vi "Find Subaddress.vi"(8 "error in":errorcluster, 10 "terminal subaddress":u16, 11 "remote terminal in":T1 format="%.0x") -> (0 "error out":errorcluster, 2 "subaddress":T1 format="%.0x", 3 "remote terminal out":T1 format="%.0x", 4 "found?":bool)   [LabVIEW 2020, in "Ballard MIL-STD-1553 Scripting.lvlib"]
uses:
  Ballard MIL-STD-1553 Scripting.lvlib
  <vilib>/NI VeriStand/Custom Device API/Custom Device Item Ref.ctl
  <vilib>/NI VeriStand/Custom Device API/Custom Device API.lvlib
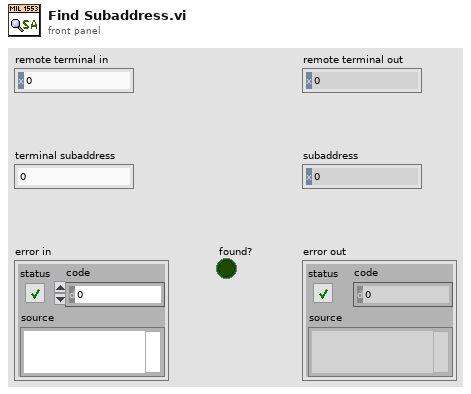
[diagram p1: front panel]
types:
  T1 = typedef "Custom Device API.lvlib/Custom Device Item Ref.ctl" = u64
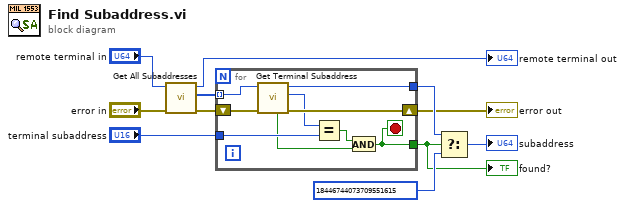
[diagram p0: block diagram]
diagram:
  n1 = call "Get All Subaddresses.vi"("error in"="error in", "remote terminal in"="remote terminal in") -> ("error out"=w6:errorcluster, "subaddresses"=w3:T1[], "remote terminal out"=→"remote terminal out":T1)  [unwired: 7 in]
  n2 = for {
    tunnel: w3 -> [w20] mode=indexing
    tunnel: "terminal subaddress" -> [w19]
    tunnel: [w14] -> w11
    tunnel: [w13] -> w2
    shift-right: [w15] -> w5
    shift-left: w6 -> [w16]
    stop <- w13 stop-if-true
    n3 = call "Get Terminal Subaddress.vi"("error in"=w16, "subaddress in"=w20) -> ("error out"=w15:errorcluster, "subaddress"=w12:u16, "subaddress out"=w14:T1, "found?"=w18:bool)  [unwired: 6 in]
    n4 = Equal?(x=w12, y=w19) -> (x = y?=w17:bool)
    n5 = And(x=w17, y=w18) -> (x .and. y?=w13:bool)
  }
  "error out" <- w5
  "found?" <- w2
  n6 = Select(t=w11, s=w2, f=T1 18446744073709551615 ("Invalid Ref")) -> (s? t:f=→"subaddress":T1)
